vi "nominal run add video.vi"(6 "out_run":i32, 7 "video_rid":string, 8 "error in (no error)":errorcluster, 9 "ref_name":string, 10 "rid":string, 11 "client":i32) -> (0 "error out":errorcluster, 3 "function return":i32, 4 "out_run out":i32)   [LabVIEW 2020, in "client.lvlib"]
doc: "int32_t nominal_run_add_video(int32_t client,\n const char *rid,\n const char *ref_name,\n const char *video_rid,\n int32_t *out_run);"
uses:
  client.lvlib
  bin/nominalClient_64.dll
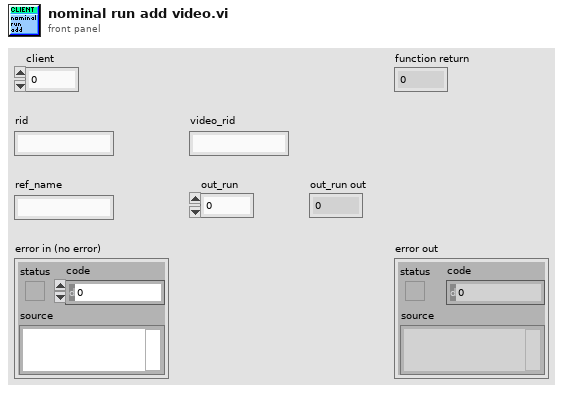
[diagram p1: front panel]
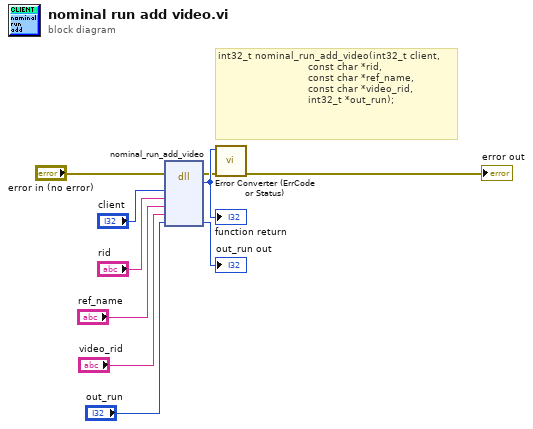
[diagram p0: block diagram]
diagram:
  # "int32_t nominal_run_add_video(int32_t client,\n                              const char *rid,\n                              const char *ref_name,\n                              const char *video_rid,\n                              int32_t *out_run);"
  n1 = dll-call lib="C:/code/labview-client-rs/lv_src/bin/nominalClient_*.*" fn="nominal_run_add_video"(error in="error in (no error)", "client"="client", "rid"="rid", "ref_name"="ref_name", "video_rid"="video_rid", "out_run"="out_run") -> (error out=w2:errorcluster, w10:i32, "out_run"=→"out_run out":i32)  [unwired: 6 in, 1 out]
  "function return" <- w10
  n2 = call "Error Converter (ErrCode or Status).vi"("error in (no error)"=w2, "error code"=w10) -> ("error out"=→"error out":errorcluster)  [unwired: 9 in]
